vi "Scoring Griddy Manipulator Controls.vi"(9 "Operator Buttons":bool[](array[boolean]), 10 "Stored Game Piece":T2=enum."Cone", 11 "Operator POVs":i16[](array[numeric])) -> (2 "Height Preset":T1=enum."High", 3 "Griddy Data":T3)   [LabVIEW 2020]
uses:
  manipulator/Implementation/Typedefs/Teleop Manipulator Commands.ctl
  manipulator/Implementation/Typedefs/game object.ctl
  manipulator/Implementation/Typedefs/Cascade Height.ctl
  <vilib>/Rock Robotics/WPI/Joystick/XBox Buttons Indexer.ctl
  9903729f-a413-4dc5-839e-aa87292b064f.vi
  e36e9bed-de20-4c5d-a46e-1ad123293361.vi
  Framework/Robot Global Data.vi
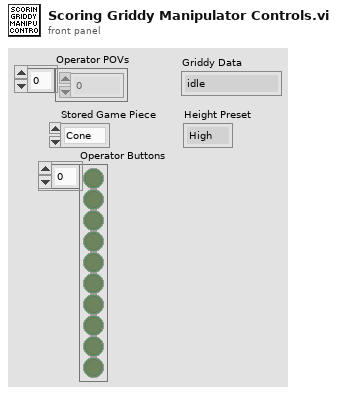
[diagram p1: front panel]
types:
  T1 = typedef "Cascade Height.ctl" = enum16{"Middle", "High"}
  T2 = typedef "game object.ctl" = enum16{"Nothing", "Cone", "Cube"}
  T3 = typedef "Teleop Manipulator Commands.ctl" = enum16{"idle", "intake cone sideways", "intake cone upright", "intake cone feeder", "intake cube feeder", "intake cube", "score low cone", "score low cube", "score mid cone", "score mid cube", "score high cone", "score high cube", "score mid cone up"}
  T4 = typedef "XBox Buttons Indexer.ctl" = enum16{"A", "B", "X", "Y", "Left Bumper", "Right Bumper", "Back", "Start", "Left Joystick", "Right Joystick"}
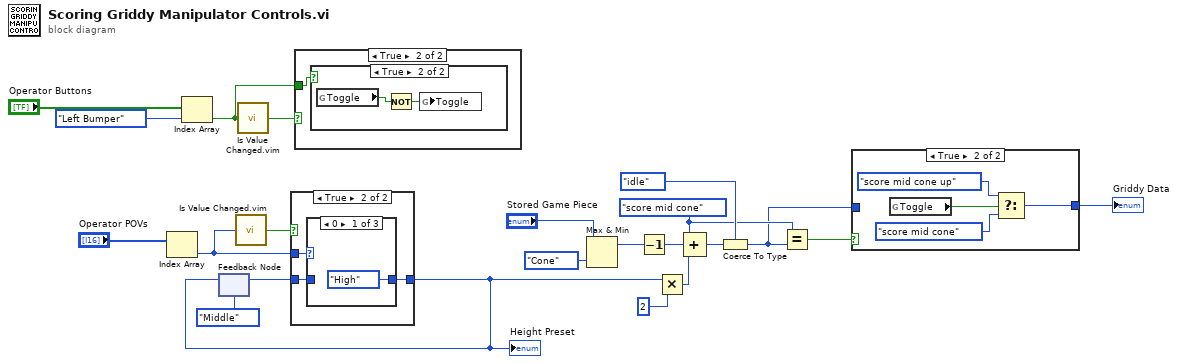
[diagram p0: block diagram]
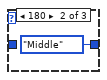
[diagram p6: hidden frame]
diagram:
  w4 = Teleop_Manipulator_Commands."score mid cone" ("y")
  n1 = Index Array(array="Operator POVs") -> (element=w22:i16)  [unwired: 1 in]
  n2 = Index Array(array="Operator Buttons", index=XBox_Buttons_Indexer."Left Bumper" ("XBox Buttons")) -> (element=w5:bool)
  n3 = feedback #1(Cascade_Height."Middle") -> (w20:T1)
  n4 = call "Is Value Changed.vim"("value"=w22) -> ("changed or first call?"=w21:bool)
  n5 = call "Is Value Changed.vim"("value"=w5) -> ("changed or first call?"=w6:bool)
  n6 = case shown="True" w21 {
    tunnel: w22 -> [_ w26]
    tunnel: w20 -> [w23 w25]
    tunnel: [w23 w24] -> w9
    frame False {
    }
    frame True {
      n7 = case shown="0" w26 {
        tunnel: w25 -> [_ _ w29]
        tunnel: [Cascade_Height."High" Cascade_Height."Middle" w29] -> w24
        frame 0 {
        }
        frame 180 {
        }
        frame -1, Default {
        }
      }
    }
  }
  "Height Preset" <- w9
  n8 = feedback-in #1(w9) -> ()
  n9 = case shown="True" w6 {
    tunnel: w5 -> [_ w30]
    frame False {
    }
    frame True {
      n10 = case shown="True" w30 {
        frame False {
        }
        frame True {
          n11 = global read "Robot Global Data.vi" "Toggle"() -> (w32:bool)
          n12 = Not(x=w32) -> (.not. x?=w31:bool)
          n13 = global write "Robot Global Data.vi" "Toggle"(w31) -> ()
        }
      }
    }
  }
  n14 = Max & Min(x="Stored Game Piece", y=game_object."Cone") -> (max(x,y)=w10:u16)  [unwired: 1 out]
  n15 = Decrement(x=w10) -> (x-1=w11:u16)
  n16 = Multiply(x=w9, y=2) -> (x*y=w17:i32)
  n17 = Compound Arithmetic op=ADD(w4, w11, w17) -> (w15:i32)
  n18 = Coerce To Type(0:w15, 1:Teleop_Manipulator_Commands."idle" ("y")) -> (2:w2:T3)
  n19 = Equal?(x=w4, y=w2) -> (x = y?=w3:bool)
  n20 = case shown="True" w3 {
    tunnel: w2 -> [w33 _]
    tunnel: [w33 w34] -> w1
    frame False {
    }
    frame True {
      n21 = global read "Robot Global Data.vi" "Toggle"() -> (w37:bool)
      n22 = Select(t=Teleop_Manipulator_Commands."score mid cone up" ("y"), s=w37, f=Teleop_Manipulator_Commands."score mid cone" ("y")) -> (s? t:f=w34:T3)
    }
  }
  "Griddy Data" <- w1
